vi "Set Output State.vi"(8 "error in (no error)":errorcluster, 10 "Output State":bool, 11 "Level Controller in":refnum<class "Level Controller.lvclass">) -> (0 "error out":errorcluster, 3 "Level Controller out":refnum<class "Level Controller.lvclass">)   [LabVIEW 2018, in "Level Controller.lvlib" / "Level Controller.lvclass"]
doc: "This VI specifies the behavior of a level controller when the variable it is monitoring goes above the deadband or below the deadband. It is only invoked in the level controller class when the operation mode switches from one mode to another. The input variable Output State is true if the current value is above the deadband and false if below the deadband."
uses:
  Level Controller.lvclass
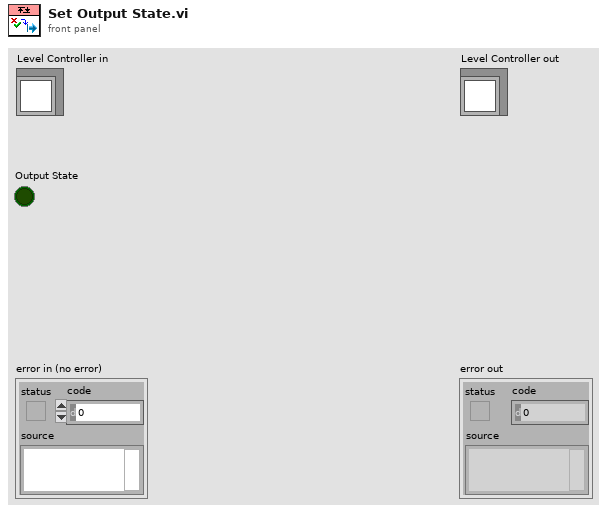
[diagram p1: front panel]
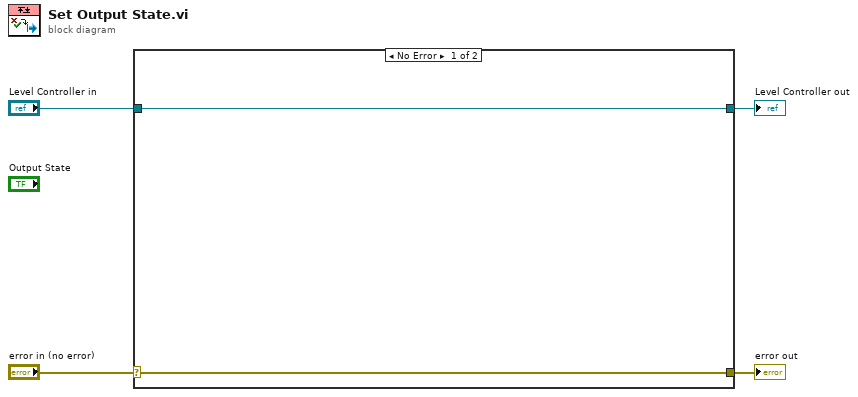
[diagram p0: block diagram]
diagram:
  n1 = case shown="No Error" "error in (no error)" {
    selector: "error in (no error)" -> [w5 w8]
    tunnel: [w5 w8] -> w3
    tunnel: [w6 w7] -> w1
    tunnel: "Level Controller in" -> [w6 w7]
    frame No Error {
    }
    frame Error {
    }
  }
  "error out" <- w3
  "Level Controller out" <- w1
